vi "lv_main.vi"   [LabVIEW 2024]
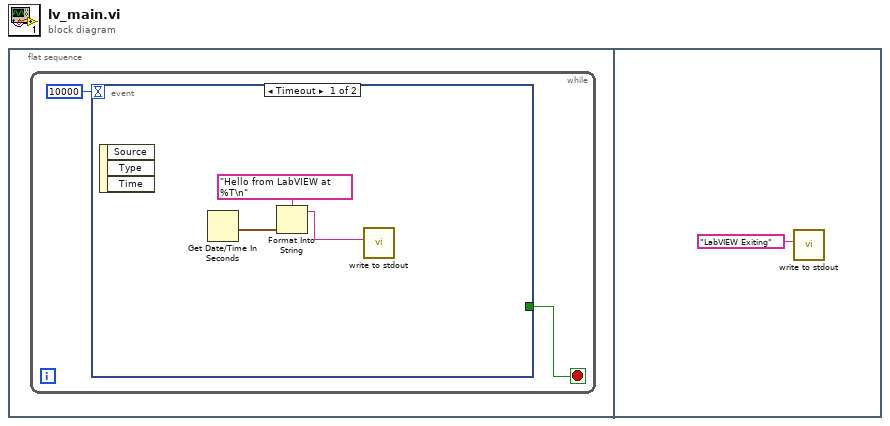
[diagram p0: block diagram]
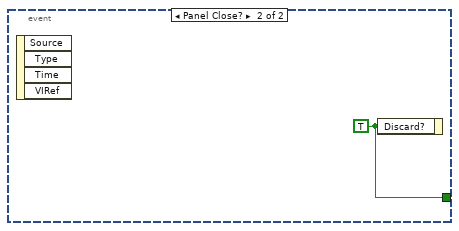
[diagram p2: hidden frame]
diagram:
  n1 = flat-sequence {
    frame #0 {
      n2 = while {
        stop <- w1 stop-if-true
        n3 = event shown="[0] Timeout" {
          selector: _ -> [_ _]
          dyn-events: _ -> [_ _]
          timeout: 10000 -> [_ _]
          tunnel: [_ w6] -> w1
          event Timeout {
            n4 = event-data() -> ()  [unwired: 1 in, 3 out]
            n5 = Get Date/Time In Seconds() -> (seconds since 1Jan1904=w3:timestamp)
            n6 = Format Into String(format string="Hello from LabVIEW at %T\n", w3) -> (resulting string=w4:string)  [unwired: 2 in, 1 out]
            n7 = call "write to stdout.vi"("data"=w4) -> ()  [unwired: 11 in]
          }
          event Panel Close? {
            w6 = TRUE ("Discard?")
            n8 = event-data() -> ()  [unwired: 1 in, 4 out]
            n9 = event-data("Discard?"=w6) -> ()  [unwired: 1 in, 1 out]
          }
        }
      }
    }
    frame #1 {
      n10 = call "write to stdout.vi"("data"="LabVIEW Exiting") -> ()  [unwired: 11 in]
    }
  }
